vi "RefNums_Actuators.vi"() -> ()   [LabVIEW 2018]
panel:
  in  "Elevator_4_PDP":i32
  out "Drive_6R":string="FrontLeftDrive"
  out "Drive_5L":string="FrontLeftDrive"
  out "Climb Foot Servo":string="FrontLeftDrive"
  in  "Elevator_3_PDP":i32
  in  "Elevator_2_PDP":i32
  in  "Elevator_1_PDP":i32
  out "Elevator_LimitSwitches":string="FrontLeftDrive"
  out "Drive_Motors":string="FrontLeftDrive"
  out "Drive_4L":string="FrontLeftDrive"
  out "Drive_3L":string="FrontLeftDrive"
  out "Lower Pulse":string="FrontLeftDrive"
  out "Lower Valve":string="FrontLeftDrive"
  out "Upper Pulse":string="FrontLeftDrive"
  out "Climber Mantis":string="FrontLeftDrive"
  out "Hatch Eject":string="FrontLeftDrive"
  out "Hatch Arm":string="FrontLeftDrive"
  out "Elevator Brake":string="FrontLeftDrive"
  out "PTO":string="FrontLeftDrive"
  out "Spare Victor":string="FrontLeftDrive"
  out "DriveSystem":string="FrontLeftDrive"
  out "Drive_2R":string="FrontLeftDrive"
  out "Drive_1R":string="FrontLeftDrive"
  out "Elevator":string="FrontLeftDrive"
  in  "Upper_Intake_PDP":i32
  in  "Lower_Intake_PDP":i32
  out "Upper_Intake":string="FrontLeftDrive"
  out "Lower_Intake":string="FrontLeftDrive"
  out "Cargo Arm":string="FrontLeftDrive"
  out "VacuumPump":string="FrontLeftDrive"
  out "Upper Valve":string="FrontLeftDrive"
  out "Shifters":string="FrontLeftDrive"
  out "ButterflyPneumatic":string="FrontLeftDrive"
  out "Compressor":string="FrontLeftDrive"
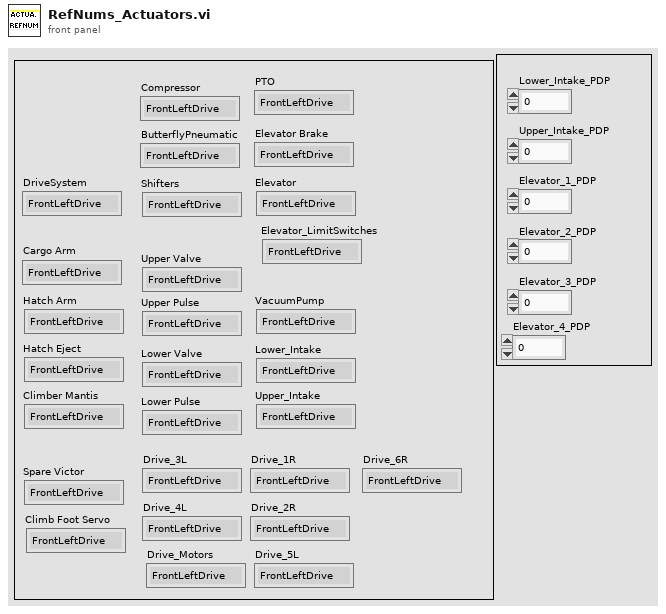
[diagram p1: front panel]
diagram:
